vi "zadanie4.vi"() -> ()   [LabVIEW 2020]
panel:
  out "Temperatura w st C obliczona na podstawie rezystancji:":dbl
  in  "Podaj wartość rezystancji opornika platynowego:":dbl
  out "Data pomiaru:":string
  out "Czas pomiaru:":string
  in  "stop":bool
  out "Podane hasło":string
  out "Podany login":string
  # "Program oblicza temperaturę w st C zmierzoną przy pomocy opornika platynowego (na podstawie jego rezystancji)"
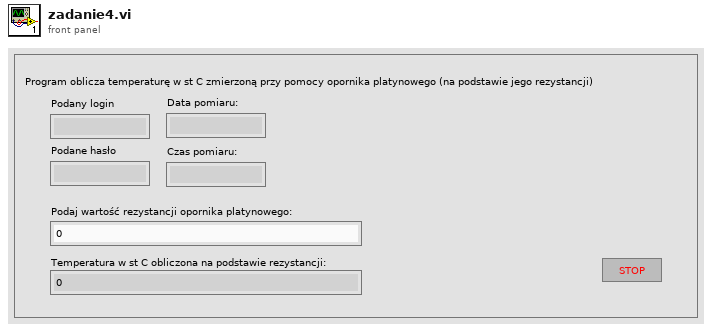
[diagram p1: front panel]
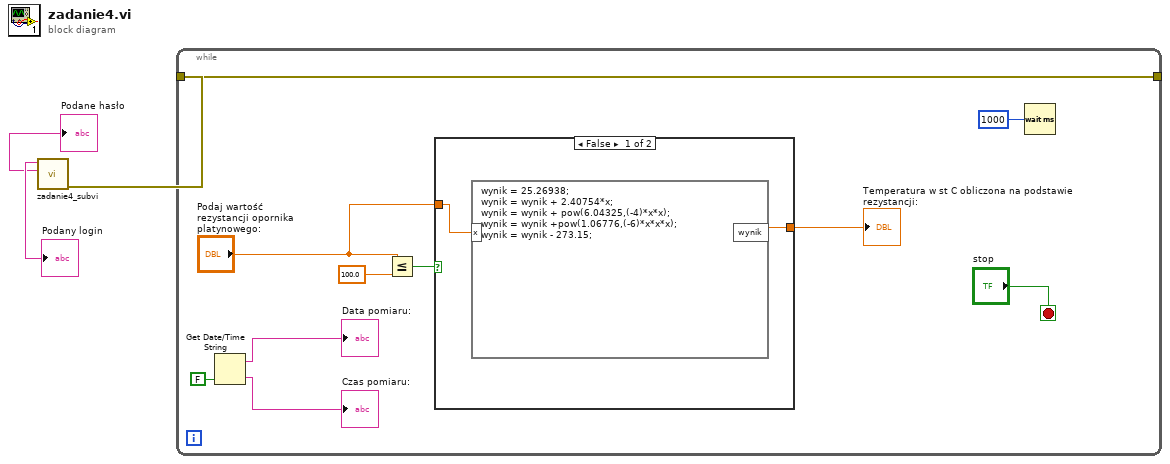
[diagram p0: block diagram]
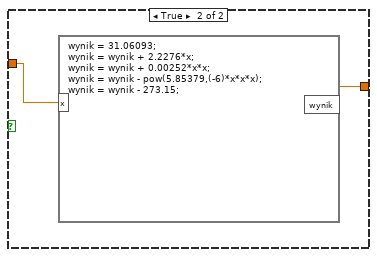
[diagram p2: hidden frame]
diagram:
  n1 = call "zadanie4_subvi.vi"() -> ("error out"=w1:errorcluster, "hasło:out"=→"Podane hasło":string, "login:out"=→"Podany login":string)  [unwired: 9 in]
  n2 = while {
    tunnel: w1 -> [w11]
    tunnel: [w11] -> _
    stop <- "stop" stop-if-true
    n3 = Get Date/Time String(want seconds? (F)=FALSE) -> (date string=→"Data pomiaru:":string, time string=→"Czas pomiaru:":string)  [unwired: 2 in]
    n4 = Less Or Equal?(x="Podaj wartość rezystancji opornika platynowego:", y=100.0) -> (x <= y?=w8:bool)
    n5 = case shown="False" w8 {
      tunnel: "Podaj wartość rezystancji opornika platynowego:" -> [w14 w16]
      tunnel: [w15 w17] -> w10
      frame False {
        n6 = formula code="wynik = 25.26938;\nwynik = wynik + 2.40754*x;\nwynik = wynik + pow(6.04325,(-4)*x*x);\nwynik = wynik +pow(1.06776,(-6)*x*x*x);\nwynik = wynik - 273.15;"("x"=w14) -> ("wynik"=w15:dbl)
      }
      frame True {
        n7 = formula code="wynik = 31.06093;\nwynik = wynik + 2.2276*x;\nwynik = wynik + 0.00252*x*x;\nwynik = wynik - pow(5.85379,(-6)*x*x*x);\nwynik = wynik - 273.15;"("x"=w16) -> ("wynik"=w17:dbl)
      }
    }
    "Temperatura w st C obliczona na podstawie rezystancji:" <- w10
    n8 = Wait (ms)(milliseconds to wait=u32 1000) -> ()  [unwired: 1 out]
  }
